vi "Subvi Get XP Environment Variables.vi"(0 "Environment Variable":string="%username%") -> (1 "Value":string, 2 "error out":errorcluster)   [LabVIEW 2012]
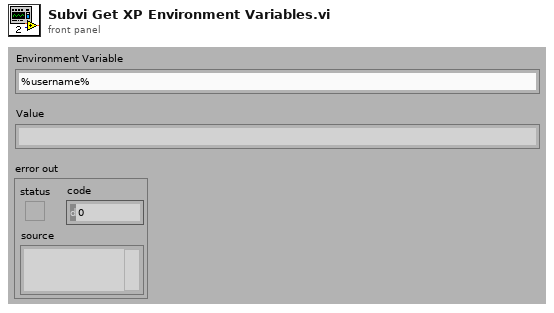
[diagram p1: front panel]
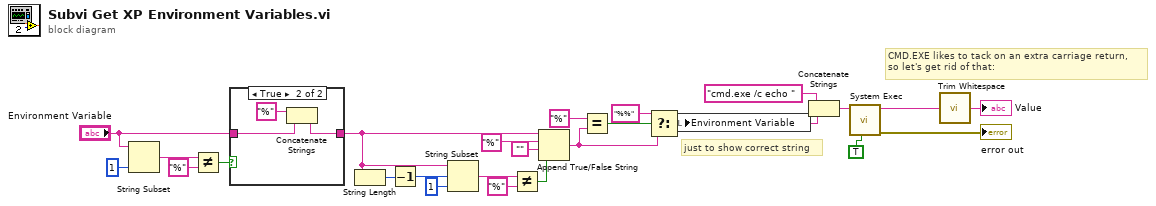
[diagram p0: block diagram]
diagram:
  # "just to show correct string"
  # "CMD.EXE likes to tack on an extra carriage return,\nso let's get rid of that:"
  n1 = String Subset(string="Environment Variable", length (rest)=1 ("length (rest)")) -> (substring=w24:string)  [unwired: 1 out]
  n2 = Not Equal?(x=w24, y="%") -> (x != y?=w22:bool)
  n3 = case shown="True" w22 {
    tunnel: "Environment Variable" -> [w26 w28]
    tunnel: [w26 w27] -> w5
    frame False {
    }
    frame True {
      n4 = Concatenate Strings("%" ("string"), w28) -> (w27:string)
    }
  }
  n5 = String Length(string=w5) -> (length=w16:i32)
  n6 = Decrement(x=w16) -> (x-1=w17:i32)
  n7 = String Subset(string=w5, offset (0)=w17, length (rest)=1 ("length (rest)")) -> (substring=w19:string)
  n8 = Not Equal?(x=w19, y="%") -> (x != y?=w4:bool)
  n9 = Append True/False String(1:w4, 2:"", 3:"%" ("string"), 4:w5) -> (0:w1:string)
  n10 = Equal?(x="%" ("y"), y=w1) -> (x = y?=w8:bool)
  n11 = Select(t="%%" ("Environment Variable"), s=w8, f=w1) -> (s? t:f=w6:string)
  n12 = local write "Environment Variable"(w6) -> ()
  n13 = Concatenate Strings("cmd.exe /c echo " ("command line"), w6) -> (w12:string)
  n14 = call <vilib>:"System Exec.vi"("run minimized? (F)"=TRUE, "command line"=w12) -> ("error out"=→"error out":errorcluster, "standard output"=w10:string)  [unwired: 4 in, 4 out]
  n15 = call <vilib>:"Trim Whitespace.vi"("string"=w10) -> ("trimmed string"=→"Value":string)  [unwired: 1 in]
